vi "Mouse Down (Deprecated).vi"(7 "Map Model in":refnum<class "Map Model.lvclass">, 8 "error in (no error)":errorcluster, 10 "Position":T1, 11 "Eraser in":refnum<class "Eraser.lvclass">) -> (0 "error out":errorcluster, 3 "Eraser out":refnum<class "Eraser.lvclass">, 5 "Map Model out":refnum<class "Map Model.lvclass">)   [LabVIEW 2020, in "Map Model.lvlib" / "Eraser.lvclass"]
uses:
  Eraser.lvclass
  <vilib>/Utility/miscctls.llb/LVPoint32TypeDef.ctl
  Map Model/Map Model.lvclass
  Undoable Tool/Undoable Tool.lvclass
  E:/Project/Labview-Projects/Completed projects/Map Editor/Models/Map Model/Tools/Undoable Tool/Undoable Tool.lvclass
panel:
  # "NOTICE -- YOU MUST LEAVE THIS NOTICE IN PLACE.\n\nCopyright (c) 2017, LIANG LIU Shawn.Liu.cn@gmail.com\nAll rights reserved.\n\nRedistribution and use in source and binary forms, with or without modification, are permitted provided that the following conditions are met:\n-Redistributions of source code must retain the above copyright notice, this list of conditions and the following disclaimer.\n-Redistributions in binary form must reproduce the above copyright notice, this list of conditions and the following disclaimer in the documentation and/or other materials provided with the distribution.\n-Neither the name of the eLp nor the names of its contributors may be used to endorse or promote products derived from this software without specific prior written permission.\n\nTHIS SOFTWARE IS PROVIDED BY THE COPYRIGHT HOLDERS AND CONTRIBUTORS \"AS IS\" AND ANY EXPRESS OR IMPLIED WARRANTIES, INCLUDING, BUT NOT LIMITED TO, THE IMPLIED WARRANTIES OF MERCHANTABILITY AND FITNESS FOR A PARTICULAR PURPOSE ARE DISCLAIMED. IN NO EVENT SHALL THE COPYRIGHT HOLDER OR CONTRIBUTORS BE LIABLE FOR ANY DIRECT, INDIRECT, INCIDENTAL, SPECIAL, EXEMPLARY, OR CONSEQUENTIAL DAMAGES (INCLUDING, BUT NOT LIMITED TO, PROCUREMENT OF SUBSTITUTE GOODS OR SERVICES; LOSS OF USE, DATA, OR PROFITS; OR BUSINESS INTERRUPTION) HOWEVER CAUSED AND ON ANY THEORY OF LIABILITY, WHETHER IN CONTRACT, STRICT LIABILITY, OR TORT (INCLUDING NEGLIGENCE OR OTHERWISE) ARISING IN ANY WAY OUT OF THE USE OF THIS SOFTWARE, EVEN IF ADVISED OF THE POSSIBILITY OF SUCH DAMAGE."
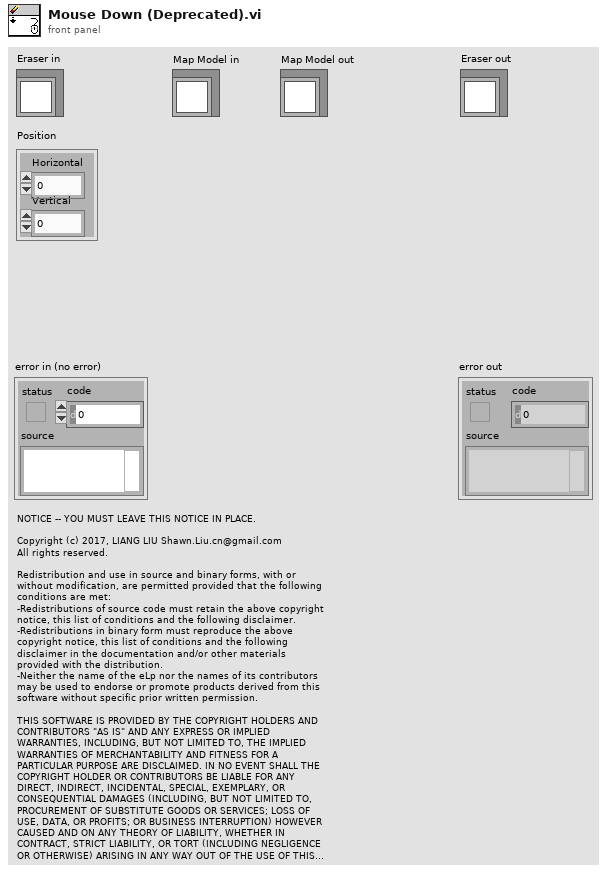
[diagram p1: front panel]
types:
  T1 = typedef "LVPoint32TypeDef.ctl" = cluster{"Horizontal":i32, "Vertical":i32}
  T2 = cluster{"Width":u16, "Style":enum32{"Solid", "Dash", "Dot", "DashDot", "DashDotDot"}}
  T3 = cluster{"Occupied Color":cluster{"Value":u8, "Color":u32}, "Free Color":cluster{"Value":u8, "Color":u32}, "Unknown Color":cluster{"Value":u8, "Color":u32}}
  T4 = typedef "LVPointTypeDef.ctl" = cluster{"Horizontal":i16, "Vertical":i16}
  T5 = typedef "imagedata.ctl" = cluster{"image type":i32, "image depth":i32, "image":u8[], "mask":u8[], "colors":u32[], "Rectangle":cluster{"left":i16, "top":i16, "right":i16, "bottom":i16}}
  T6 = cluster{"left":i16, "top":i16, "right":i16, "bottom":i16}
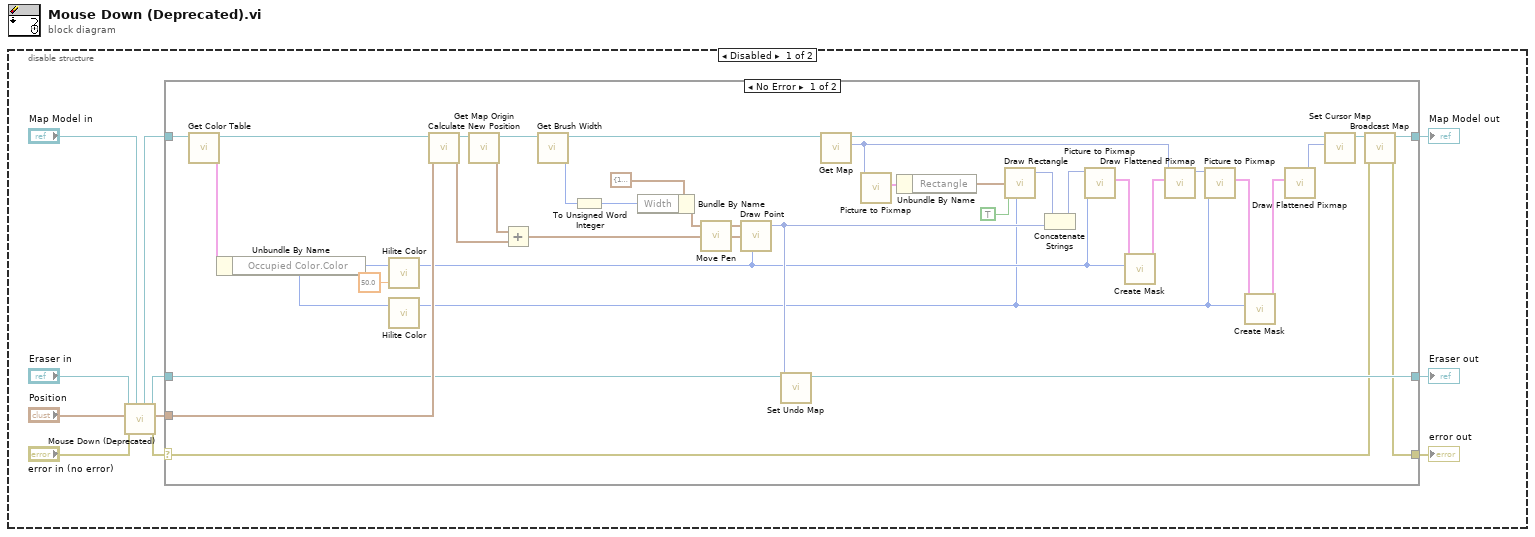
[diagram p0: block diagram]
diagram:
  n1 = disable-structure shown="Disabled" {
    frame Disabled {
      n2 = call-parent "Mouse Down (Deprecated).vi"("Map Model in"="Map Model in", "error in (no error)"="error in (no error)", "Position"="Position", "Tool in"="Eraser in") -> ("error out"=w3:errorcluster, "Tool out"=w5:refnum<class "Eraser.lvclass">, "Map Model out"=w4:refnum<class "Map Model.lvclass">)  [unwired: 5 in]
      n3 = case shown="No Error" w3 {
        selector: w3 -> [w14 w52]
        tunnel: [w49 w50] -> w10
        tunnel: "Position" -> [w48 _]
        tunnel: w5 -> [w47 w50]
        tunnel: w4 -> [w33 w51]
        tunnel: [w13 w52] -> w2
        tunnel: [w12 w51] -> w1
        frame No Error {
          n4 = call "Get Color Table.vi"("Map Model in"=w33) -> ("Color Table"=w36:T3, "Map Model out"=w32:refnum<class "Map Model.lvclass">)  [unwired: 9 in]
          n5 = Unbundle By Name(w36) -> ("Occupied Color.Color"=w34:u32)
          n6 = call <vilib>:"Hilite Color.vi"("Percentage(30)"=50.0, "Color In"=w34) -> ("Hilite"=w16:u32)  [unwired: 1 out]
          n7 = call <vilib>:"Hilite Color.vi"("Color In"=w34) -> ("Hilite"=w15:u32)  [unwired: 1 in, 1 out]
          n8 = call "Calculate New Position.vi"("Position in"=w48, "Map Model in"=w32) -> ("Position out"=w44:T1, "Map Model out"=w45:refnum<class "Map Model.lvclass">)  [unwired: 8 in]
          n9 = call "Get Map Origin.vi"("Map Model in"=w45) -> ("Map Origin"=w46:T4, "Map Model out"=w40:refnum<class "Map Model.lvclass">)  [unwired: 9 in]
          n10 = Add(x=w46, y=w44) -> (x+y=w38:T1)
          n11 = call "Get Brush Width.vi"("Map Model in"=w40) -> ("Brush Width"=w42:i32, "Map Model out"=w18:refnum<class "Map Model.lvclass">)  [unwired: 9 in]
          n12 = To Unsigned Word Integer(number=w42) -> (unsigned 16bit integer=w41:u16)
          n13 = Bundle By Name(cluster=T2 {"Width"=1, "Style"=enum."Solid"} ("pen"), "Width"=w41) -> (w39:T2)
          n14 = call <vilib>:"Move Pen.vi"("new position"=w38) -> ("new picture"=w37:picture)  [unwired: 4 in]
          n15 = call <vilib>:"Draw Point.vi"("picture"=w37, "point(x,y)"=w38, "color(black)"=w16, "pen"=w39) -> ("new picture"=w17:picture)  [unwired: 5 in]
          n16 = call "Set Undo Map.vi"("Undo Map"=w17, "Undoable Tool in"=w47) -> ("Undoable Tool out"=w49:refnum<class "Eraser.lvclass">)  [unwired: 9 in]
          n17 = call "Get Map.vi"("Map Model in"=w18) -> ("Map"=w11:picture, "Map Model out"=w30:refnum<class "Map Model.lvclass">)  [unwired: 9 in]
          n18 = call <vilib>:"Picture to Pixmap.vi"("picture"=w11) -> ("image data"=w29:T5)  [unwired: 9 in, 1 out]
          n19 = Unbundle By Name(w29) -> ("Rectangle"=w28:T6)
          n20 = call <vilib>:"Draw Rectangle.vi"("rect"=w28, "fill?(F)"=TRUE, "color(black)"=w15) -> ("new picture"=w27:picture)  [unwired: 6 in]
          n21 = Concatenate Strings(w27, w17) -> (w21:picture)
          n22 = call <vilib>:"Picture to Pixmap.vi"("Background Color"=w16, "picture"=w21) -> ("image data"=w26:T5)  [unwired: 8 in, 1 out]
          n23 = call <vilib>:"Create Mask.vi"("Mask Color (Black)"=w16, "image data"=w26) -> ("image data"=w25:T5)  [unwired: 9 in]
          n24 = call <vilib>:"Draw Flattened Pixmap.vi"("image data"=w25, "picture"=w11) -> ("new picture"=w22:picture)  [unwired: 7 in]
          n25 = call <vilib>:"Picture to Pixmap.vi"("Background Color"=w15, "picture"=w22) -> ("image data"=w23:T5)  [unwired: 8 in, 1 out]
          n26 = call <vilib>:"Create Mask.vi"("Mask Color (Black)"=w15, "image data"=w23) -> ("image data"=w24:T5)  [unwired: 9 in]
          n27 = call <vilib>:"Draw Flattened Pixmap.vi"("image data"=w24) -> ("new picture"=w19:picture)  [unwired: 8 in]
          n28 = call "Set Cursor Map.vi"("Cursor Map"=w19, "Map Model in"=w30) -> ("Map Model out"=w31:refnum<class "Map Model.lvclass">)  [unwired: 9 in]
          n29 = call "Broadcast Map.vi"("error in (no error)"=w14, "Map Model in"=w31) -> ("error out"=w13:errorcluster, "Map Model out"=w12:refnum<class "Map Model.lvclass">)  [unwired: 8 in]
        }
        frame Error {
        }
      }
      "error out" <- w2
      "Eraser out" <- w10
      "Map Model out" <- w1
    }
    frame Enabled {
    }
  }
